vi "Write Register.vi"(7 "Unit ID (A)":string="A", 8 "error in":errorcluster, 9 "Register Value":i32 format="%.0x", 10 "Register address":u16, 11 "VISA Session In":refnum<visa-resource-name>="Alicat") -> (0 "error out":errorcluster, 2 "Register Written Successfully":bool, 3 "VISA Session Out":refnum<visa-resource-name>)   [LabVIEW 2015]
doc: "Writes the specified integer value into the desired configuration register of an Alicat device."
uses:
  <vilib>/Instr/_visa.llb/VISA Flush IO Buffer Mask.ctl
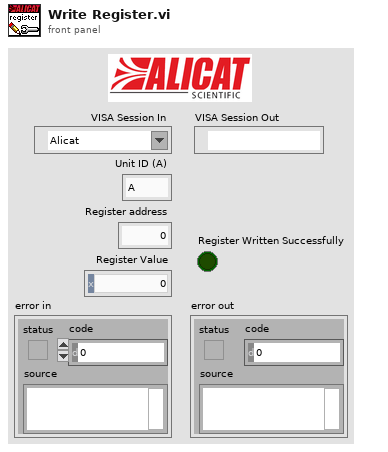
[diagram p1: front panel]
types:
  T1 = typedef "VISA Flush IO Buffer Mask.ctl" = u16
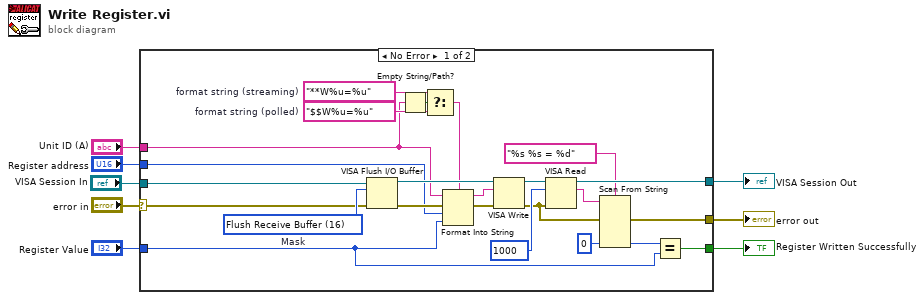
[diagram p0: block diagram]
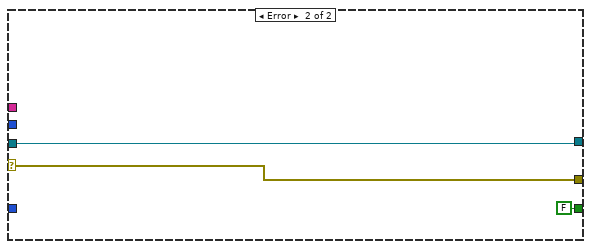
[diagram p2: hidden frame]
diagram:
  n1 = case shown="No Error" "error in" {
    selector: "error in" -> [w17 w35]
    tunnel: [w29 w34] -> w8
    tunnel: [w12 w35] -> w7
    tunnel: "Register address" -> [w24 _]
    tunnel: "Register Value" -> [w10 _]
    tunnel: "Unit ID (A)" -> [w20 _]
    tunnel: "VISA Session In" -> [w18 w34]
    tunnel: [w9 FALSE] -> w1
    frame No Error {
      w21 = "**W%u=%u"  # format string (streaming)
      w23 = "$$W%u=%u"  # format string (polled)
      w31 = T1 16 items=["Flush Receive Buffer"=16, "Write Transmit Buffer to Device"=32, "Flush Receive Buffer (No I/O)"=64, "Flush Transmit Buffer"=128]  # Mask
      n2 = VISA Flush I/O Buffer(VISA resource name=w18, mask (16)=w31, error in (no error)=w17) -> (VISA resource name out=w32:refnum<visa-resource-name>, error out=w26:errorcluster)
      n3 = Empty String/Path?(string/path=w20) -> (empty?=w22:bool)
      n4 = Select(t=w21, s=w22, f=w23) -> (s? t:f=w19:string)
      n5 = Format Into String(format string=w19, initial string=w20, error in=w26, w24, w10) -> (resulting string=w27:string, error out=w25:errorcluster)
      n6 = VISA Write(VISA resource name=w32, write buffer=w27, error in (no error)=w25) -> (VISA resource name out=w30:refnum<visa-resource-name>, error out=w13:errorcluster)  [unwired: 1 out]
      n7 = VISA Read(VISA resource name=w30, byte count=u32 1000, error in (no error)=w13) -> (VISA resource name out=w29:refnum<visa-resource-name>, read buffer=w16:string)  [unwired: 2 out]
      n8 = Scan From String(format string="%s %s = %d", input string=w16, error in=w13, default 3=0 ("default value 3")) -> (error out=w12:errorcluster, output 3=w11:i32)  [unwired: 5 in, 2 out]
      n9 = Equal?(x=w11, y=w10) -> (x = y?=w9:bool)
    }
    frame Error {
    }
  }
  "error out" <- w7
  "VISA Session Out" <- w8
  "Register Written Successfully" <- w1
